vi "FileIO_GetMostRecentPathBySize.vi"(0 "Path In":path, 5 "File or Folder ?":enum16{"Folder", "File"}(ring)=enum."File", 7 "Size Limit":i64, 9 "Comparison":enum16{"LT <", "GT >"}(ring)=enum."GT >", 11 "Error In":errorcluster) -> (4 "Path Out":path, 6 "Found ?":bool, 8 "Report Text":string, 15 "Error Out":errorcluster)   [LabVIEW 2016]
doc: "This VI will search and return the file/folder path for the most recent (newest) file/folder that is greater than or less than a particular file size from within a given folder. If folder is empty returns empty path.\n\nAlso returns a boolean for whether or not most recent file/folder is found, along with report text if folder was empty."
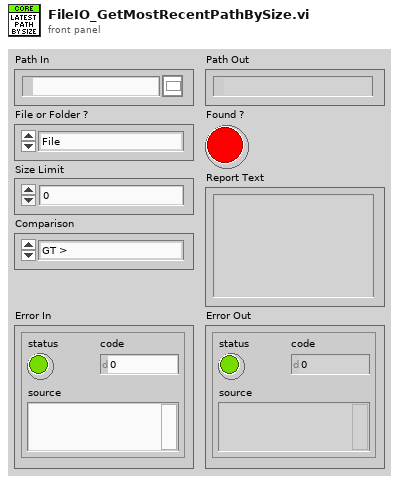
[diagram p1: front panel]
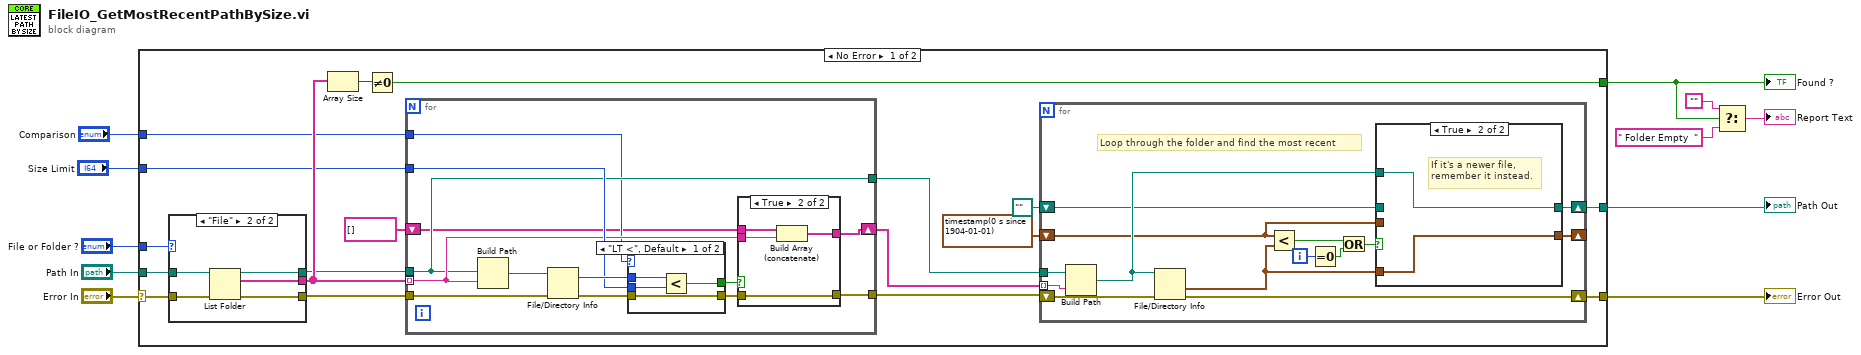
[diagram p0: block diagram]
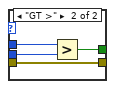
[diagram p2: hidden frame]
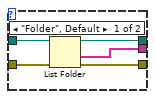
[diagram p4: hidden frame]
diagram:
  n1 = case shown="No Error" "Error In" {
    selector: "Error In" -> [w25 w85]
    tunnel: [w29 w85] -> w8
    tunnel: "Path In" -> [w24 _]
    tunnel: [w26 _] -> w7
    tunnel: "File or Folder ?" -> [w23 _]
    tunnel: [w21 _] -> w6
    tunnel: "Size Limit" -> [w17 _]
    tunnel: "Comparison" -> [w14 _]
    frame No Error {
      n2 = case shown="\"File\"" w23 {
        tunnel: [w57 w62] -> w20
        tunnel: [w60 w66] -> w18
        tunnel: w24 -> [w61 w65]
        tunnel: w25 -> [w59 w64]
        tunnel: [w58 w63] -> w19
        frame "Folder", Default {
          n3 = List Folder(path=w61, error in=w59) -> (path out=w60:path, folder names=w57:string[], error out=w58:errorcluster)  [unwired: 2 in, 1 out]
        }
        frame "File" {
          n4 = List Folder(path=w65, error in=w64) -> (path out=w66:path, filenames=w62:string[], error out=w63:errorcluster)  [unwired: 2 in, 1 out]
        }
      }
      n5 = Array Size(array=w20) -> (size(s)=w22:i32)
      n6 = Not Equal To 0?(x=w22) -> (x != 0?=w21:bool)
      n7 = for {
        tunnel: w20 -> [w37] mode=indexing
        tunnel: w19 -> [w42]
        tunnel: w18 -> [w35]
        tunnel: w17 -> [w39]
        tunnel: [w36] -> w16
        tunnel: [w35] -> w15
        tunnel: w14 -> [w34]
        shift-right: [w31] -> w12
        shift-left: string[] [] -> [w30]
        n8 = Build Path(base path=w35, name or relative path=w37) -> (appended path=w41:path)
        n9 = File/Directory Info(path=w41, error in=w42) -> (size=w40:i64, error out=w33:errorcluster)  [unwired: 5 out]
        n10 = case shown="\"LT <\", Default" w34 {
          tunnel: w40 -> [w46 w50]
          tunnel: w39 -> [w45 w49]
          tunnel: [w44 w48] -> w38
          tunnel: w33 -> [w43 w47]
          tunnel: [w43 w47] -> w32
          frame "LT <", Default {
            n11 = Less?(x=w46, y=w45) -> (x < y?=w44:bool)
          }
          frame "GT >" {
            n12 = Greater?(x=w50, y=w49) -> (0:w48:bool)
          }
        }
        n13 = case shown="True" w38 {
          tunnel: w37 -> [_ w55]
          tunnel: w32 -> [w52 w56]
          tunnel: [w52 w56] -> w36
          tunnel: [w51 w54] -> w31
          tunnel: w30 -> [w51 w53]
          frame False {
          }
          frame True {
            n14 = Build Array (concatenate)(w53, w55) -> (w54:string[])
          }
        }
      }
      n15 = for {
        shift-right: [w75] -> _
        shift-left: timestamp(0 s since 1904-01-01) ("last mod 2") -> [w68]
        shift-right: [w73] -> w26
        shift-left: path "" -> [w72]
        shift-right: [w71] -> w29
        shift-left: w16 -> [w80]
        tunnel: w15 -> [w70]
        tunnel: w12 -> [w67] mode=indexing
        i -> [w76]
        # "Loop through the folder and find the most recent"
        n16 = Build Path(base path=w70, name or relative path=w67) -> (appended path=w74:path)
        n17 = File/Directory Info(path=w74, error in=w80) -> (last mod=w69:timestamp, error out=w71:errorcluster)  [unwired: 5 out]
        n18 = Less?(x=w68, y=w69) -> (x < y?=w78:bool)
        n19 = Equal To 0?(x=w76) -> (x = 0?=w77:bool)
        n20 = Or(x=w78, y=w77) -> (x .or. y?=w79:bool)
        n21 = case shown="True" w79 {
          tunnel: w68 -> [w82 _]
          tunnel: [w82 w84] -> w75
          tunnel: w69 -> [_ w84]
          tunnel: w74 -> [_ w83]
          tunnel: [w81 w83] -> w73
          tunnel: w72 -> [w81 _]
          frame False {
          }
          frame True {
            # "If it's a newer file,\nremember it instead."
          }
        }
      }
    }
    frame Error {
    }
  }
  "Found ?" <- w6
  "Path Out" <- w7
  "Error Out" <- w8
  n22 = Select(t="", s=w6, f=" Folder Empty  ") -> (s? t:f=→"Report Text":string)
